vi "Simple Reader.vi"(8 "error in (no error)":errorcluster, 11 "LakeShore T Controller Driver in":refnum<class "LakeShore T Controller Driver.lvclass">) -> (0 "error out":errorcluster, 2 "Signals":dbl[](array[numeric]), 3 "LakeShore T Controller Driver out":refnum<class "LakeShore T Controller Driver.lvclass">)   [LabVIEW 2016, in "LakeShore T Controller Driver.lvclass"]
uses:
  LakeShore T Controller Driver.lvclass
  C:/github/NHMFL_Core/Libraries/Instruments/VISA Instrument/VISA Instrument.lvclass
  C:/github/NHMFL_Core/Libraries/Instruments/Temperature Controller Driver/Temperature Controller Driver.lvclass
  VISA Instrument/VISA Instrument.lvclass/VISA Instrument.ctl
  VISA Instrument/Read VISA resource.vi
  VISA Instrument/Write VISA resource.vi
  Temperature Controller Driver/Read T controller configuration.vi
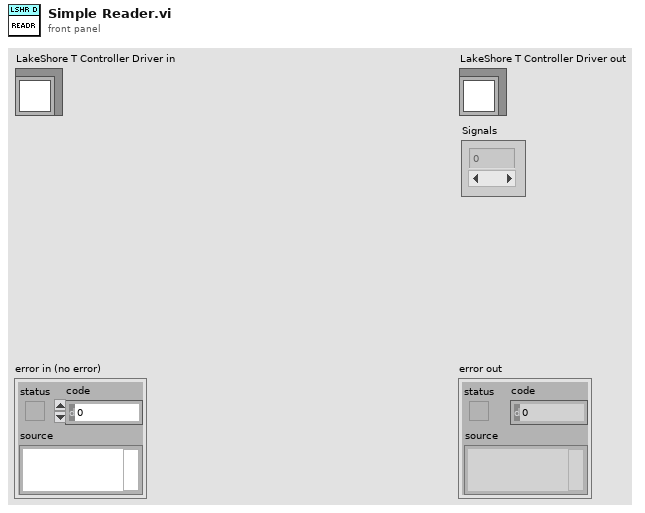
[diagram p1: front panel]
types:
  T1 = typedef "T controller configuration.ctl" = cluster{"Record Channels":string[], "Add raw signal":bool, "New set point":dbl}
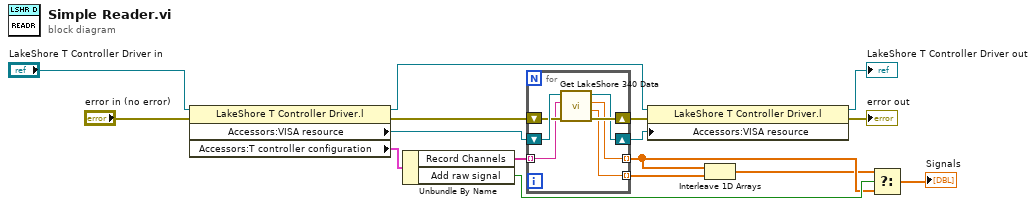
[diagram p0: block diagram]
diagram:
  n1 = property class="LakeShore T Controller Driver.l"(reference="LakeShore T Controller Driver in", error in="error in (no error)") -> (reference out=w14:refnum<class "LakeShore T Controller Driver.lvclass">, error out=w13:errorcluster, "Accessors:VISA resource"=w12:refnum<visa-resource-name>, "Accessors:T controller configuration"=w11:T1)
  n2 = Unbundle By Name(w11) -> ("Record Channels"=w10:string[], "Add raw signal"=w5:bool)
  n3 = for {
    tunnel: w10 -> [w19] mode=indexing
    shift-right: [w21] -> w16
    shift-left: w13 -> [w22]
    shift-right: [w20] -> w15
    shift-left: w12 -> [w23]
    tunnel: [w18] -> w4 mode=indexing
    tunnel: [w17] -> w3 mode=indexing
    n4 = call "Get LakeShore 340 Data.vi"("error in (no error)"=w22, "Input (A or B)"=w19, "VISA Resource Name"=w23) -> ("error out"=w21:errorcluster, "Raw"=w17:dbl, "Temperature"=w18:dbl, "VISA Resource Name Out"=w20:refnum<visa-resource-name>)  [unwired: 5 in]
  }
  n5 = property class="LakeShore T Controller Driver.l"(reference=w14, error in=w16, "Accessors:VISA resource"=w15) -> (reference out=→"LakeShore T Controller Driver out":refnum<class "LakeShore T Controller Driver.lvclass">, error out=→"error out":errorcluster)
  n6 = Interleave 1D Arrays(w4, w3) -> (w2:dbl[])
  n7 = Select(t=w2, s=w5, f=w4) -> (s? t:f=→"Signals":dbl[])
